vi "IncOrDecList.vi"(7 "Step Size?":i32, 9 "Input":dbl, 10 "Vals":dbl[](array[numeric]), 11 "Shift":bool) -> (3 "Output":dbl)   [LabVIEW 2022 SP3]
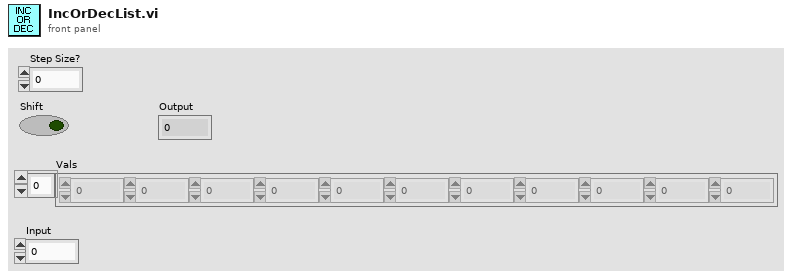
[diagram p1: front panel]
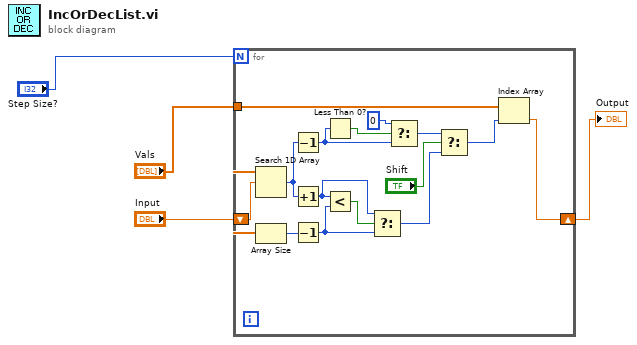
[diagram p0: block diagram]
diagram:
  n1 = for {
    N: "Step Size?" -> [_]
    tunnel: "Vals" -> [w18]
    shift-right: [w5] -> w1
    shift-left: "Input" -> [w19]
    n2 = Search 1D Array(1D array=w18, element=w19) -> (index of element=w7:i32)  [unwired: 1 in]
    n3 = Array Size(array=w18) -> (size(s)=w17:i32)
    n4 = Decrement(x=w7) -> (x-1=w14:i32)
    n5 = Increment(x=w7) -> (x+1=w6:i32)
    n6 = Decrement(x=w17) -> (x-1=w8:i32)
    n7 = Less Than 0?(x=w14) -> (x < 0?=w13:bool)
    n8 = Less?(x=w6, y=w8) -> (x < y?=w16:bool)
    n9 = Select(t=w6, s=w16, f=w8) -> (s? t:f=w15:i32)
    n10 = Select(t=0, s=w13, f=w14) -> (s? t:f=w12:i32)
    n11 = Select(t=w12, s="Shift", f=w15) -> (s? t:f=w10:i32)
    n12 = Index Array(array=w18, index=w10) -> (element=w5:dbl)
  }
  "Output" <- w1
